vi "channel operation tests.vi"() -> ()   [LabVIEW 2013, in "processing plugin tests.lvlib"]
uses:
  processing plugin tests.lvlib
  module/configuration/tag bus processing plugin module configuration.lvclass
  <vilib>/NI/Tag Bus Module Framework/channel/TBM channel.lvclass
panel:
  out "channels match":bool
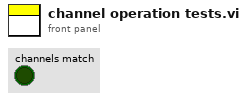
[diagram p1: front panel]
types:
  T1 = typedef "tag bus processing plugin module configuration.lvclass/processing channels.ctl" = cluster{"parameter":refnum<class "TBM channel.lvclass">, "result":refnum<class "TBM channel.lvclass">}
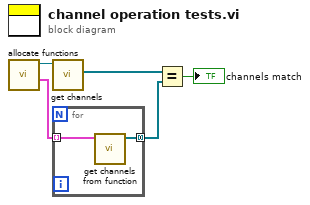
[diagram p0: block diagram]
diagram:
  n1 = call "allocate functions.vi"() -> ("functions"=w2:T1[], "tag bus processing plugin module configuration out"=w3:refnum<class "tag bus processing plugin module configuration.lvclass">)  [unwired: 9 in, 1 out]
  n2 = call-dynamic "get channels.vi"("module configuration in"=w3) -> ("channels"=w5:refnum<class "TBM channel.lvclass">[])  [unwired: 9 in, 1 out]
  n3 = for {
    tunnel: w2 -> [w7] mode=indexing
    tunnel: [w6] -> w1 mode=concatenating
    n4 = call "get channels from function.vi"("processing function"=w7) -> ("channels"=w6:refnum<class "TBM channel.lvclass">[])  [unwired: 10 in]
  }
  n5 = Equal?(x=w5, y=w1) -> (x = y?=→"channels match":bool)
